vi "Sequence.Compile.vi"(8 "error in (no error)":errorcluster, 11 "State Variables":T1) -> (0 "error out":errorcluster, 2 "output cluster":T3, 3 "State Variables out":T1)   [LabVIEW 2013, in "Simple Sequence Editor.lvlib"]
uses:
  Simple Sequence Editor.lvlib
  Types/StateVariables.ctl
  Types/ChannelProperties.ctl
  Types/Compiled.RTSequenceProperties.ctl
  Types/Compiled.StepProperties.ctl
  Types/Compiled.IOStateProperties.ctl
  Types/Compiled.StepElementProperties.ctl
  Types/StepTypes.ctl
  Types/Compiled.StepCondition.ctl
  Types/OperationTypes.ctl
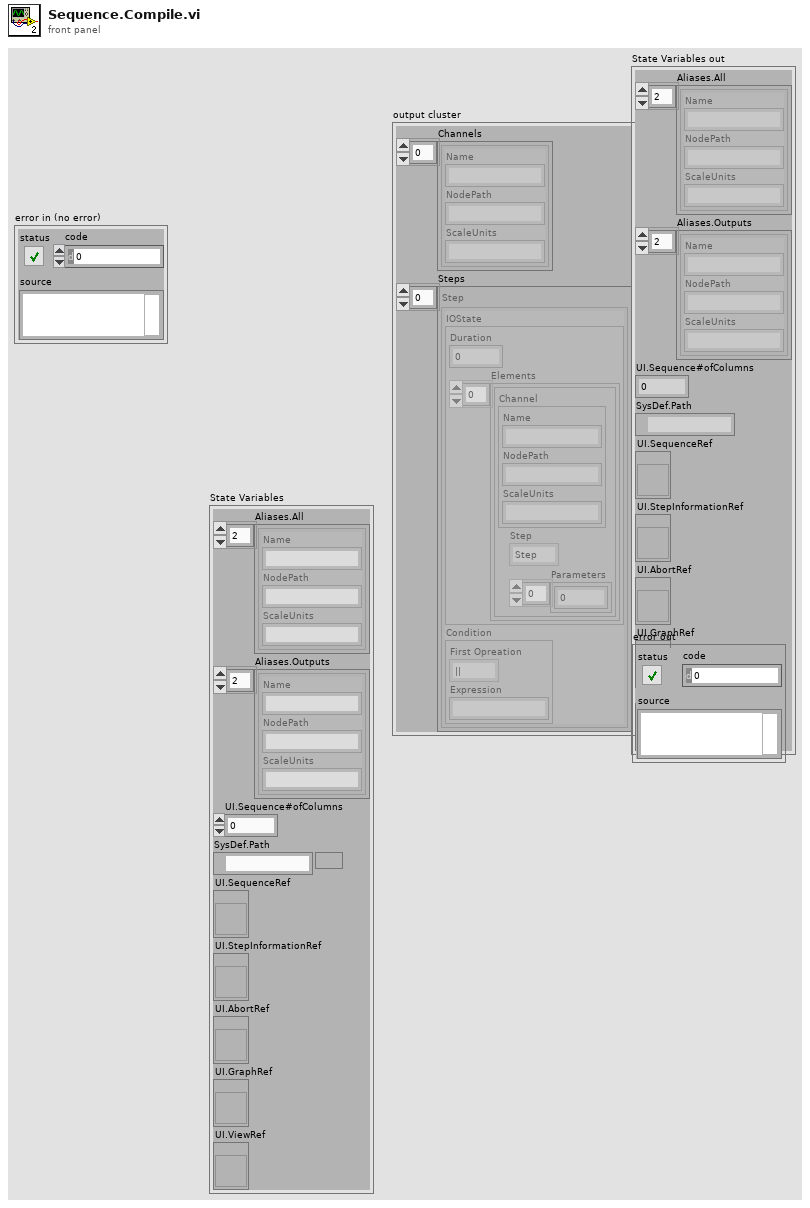
[diagram p1: front panel]
types:
  T1 = typedef "Simple Sequence Editor.lvlib/StateVariables.ctl" = cluster{"Aliases.All":T2[], "Aliases.Outputs":T2[], "UI.Sequence#ofColumns":i32, "SysDef.Path":path, "UI.SequenceRef":refnum<vi>, "UI.StepInformationRef":refnum<vi>, "UI.AbortRef":refnum<vi>, "UI.GraphRef":refnum<vi>, "UI.ViewRef":refnum<vi>}
  T2 = typedef "Simple Sequence Editor.lvlib/ChannelProperties.ctl" = cluster{"Name":string, "NodePath":string, "ScaleUnits":string}
  T3 = typedef "Simple Sequence Editor.lvlib/Compiled.RTSequenceProperties.ctl" = cluster{"Channels":T2[], "Steps":T4[]}
  T4 = typedef "Simple Sequence Editor.lvlib/Compiled.StepProperties.ctl" = cluster{"IOState":T5, "Condition":T8}
  T5 = typedef "Simple Sequence Editor.lvlib/Compiled.IOStateProperties.ctl" = cluster{"Duration":dbl, "Elements":T6[]}
  T6 = typedef "Simple Sequence Editor.lvlib/Compiled.StepElementProperties.ctl" = cluster{"Channel":T2, "Step":T7, "Parameters":dbl[]}
  T7 = typedef "Simple Sequence Editor.lvlib/StepTypes.ctl" = enum8{"Step", "iStep", "Ramp", "Unchanged", "Unknown"}
  T8 = typedef "Simple Sequence Editor.lvlib/Compiled.StepCondition.ctl" = cluster{"First Opreation":T9, "Expression":string}
  T9 = typedef "Simple Sequence Editor.lvlib/OperationTypes.ctl" = enum8{"None", "&&", "||"}
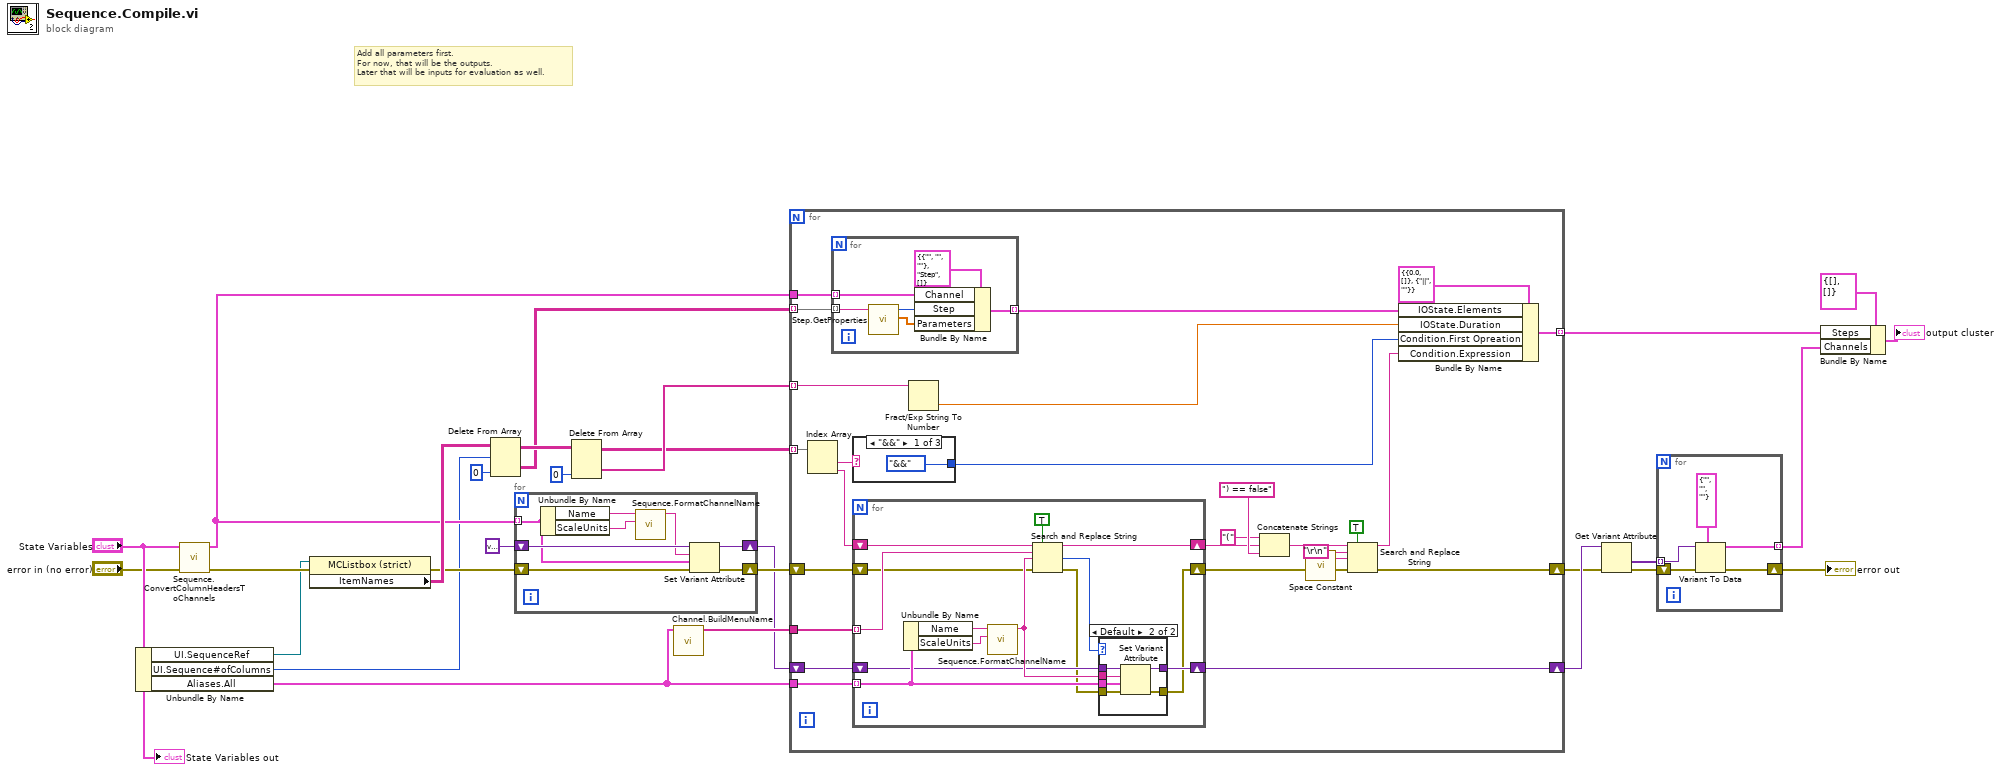
[diagram p0: block diagram]
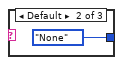
[diagram p3: hidden frame]
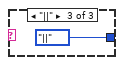
[diagram p4: hidden frame]
diagram:
  # "Add all parameters first.\nFor now, that will be the outputs.\nLater that will be inputs for evaluation as well."
  n1 = Unbundle By Name("State Variables") -> ("UI.SequenceRef"=w2:refnum<vi>, "UI.Sequence#ofColumns"=w1:i32, "Aliases.All"=w17:T2[])
  n2 = call "Sequence.ConvertColumnHeadersToChannels.vi"("error in (no error)"="error in (no error)", "State Variables"="State Variables") -> ("error out"=w3:errorcluster, "Output Channels"=w14:T2[])  [unwired: 8 in]
  n3 = property class="MCListbox (strict)"(reference=w2, error in=w3) -> (error out=w13:errorcluster, "ItemNames"=w25:string[][])  [unwired: 1 out]
  n4 = Delete From Array(array=w25, length=w1, index (col)=0 ("disabled index (col)")) -> (deleted portion=w23:string[][], array with subset deleted=w28:string[][])  [unwired: 1 in]
  n5 = for {
    shift-right: [w35] -> w11
    shift-left: variant ("variant") -> [w36]
    shift-right: [w34] -> w12
    shift-left: w13 -> [w33]
    tunnel: w14 -> [w32] mode=indexing
    n6 = Unbundle By Name(w32) -> ("Name"=w31:string, "ScaleUnits"=w30:string)
    n7 = call "Sequence.FormatChannelName.vi"("ScaleUnits"=w30, "Name"=w31) -> ("String"=w29:string)  [unwired: 9 in]
    n8 = Set Variant Attribute(Variant=w36, name=w29, value=w32, error in=w33) -> (Variant out=w35:variant, error out=w34:errorcluster)  [unwired: 1 out]
  }
  n9 = Delete From Array(array=w28, index (col)=0 ("disabled index (col)")) -> (deleted portion=w24:string[], array with subset deleted=w19:string[][])  [unwired: 2 in]
  n10 = call "Channel.BuildMenuName.vi"("Aliases"=w17) -> ("Aliases Array"=w18:string[])  [unwired: 10 in]
  n11 = for {
    tunnel: w24 -> [w62] mode=indexing
    tunnel: w23 -> [w61] mode=indexing
    tunnel: w14 -> [w60]
    tunnel: [w50] -> w21 mode=indexing
    tunnel: w19 -> [w55] mode=indexing
    tunnel: w18 -> [w54]
    tunnel: w17 -> [w53]
    shift-right: [w44] -> w8
    shift-left: w12 -> [w52]
    shift-right: [w39] -> w10
    shift-left: w11 -> [w40]
    n12 = Index Array(array=w55) -> (element #1=w56:string, element #2=w57:string)  [unwired: 2 in]
    n13 = for {
      tunnel: w61 -> [w93] mode=indexing
      tunnel: w60 -> [w91] mode=indexing
      tunnel: [w88] -> w38 mode=indexing
      n14 = call "Step.GetProperties.vi"("String in"=w93) -> ("Parameters"=w89:dbl[], "Step"=w90:T7)  [unwired: 9 in]
      n15 = Bundle By Name(cluster=T6 {"Channel"={"Name"="", "NodePath"="", "ScaleUnits"=""}, "Step"=enum."Step", "Parameters"=[]}, "Channel"=w91, "Step"=w90, "Parameters"=w89) -> (w88:T6)
    }
    n16 = case shown="\"&&\"" w56 {
      tunnel: [OperationTypes."&&" OperationTypes."None" OperationTypes."||"] -> w41
      frame "&&" {
      }
      frame Default {
      }
      frame "||" {
      }
    }
    n17 = for {
      tunnel: w54 -> [w76] mode=indexing
      tunnel: w53 -> [w70] mode=indexing
      shift-right: [w63] -> w45
      shift-left: w52 -> [w67]
      shift-right: [w71] -> w58
      shift-left: w57 -> [w75]
      shift-right: [w68] -> w39
      shift-left: w40 -> [w65]
      n18 = Unbundle By Name(w70) -> ("Name"=w73:string, "ScaleUnits"=w74:string)
      n19 = call "Sequence.FormatChannelName.vi"("ScaleUnits"=w74, "Name"=w73) -> ("String"=w69:string)  [unwired: 9 in]
      n20 = Search and Replace String(replace all?=TRUE ("replace all? (F)"), input string=w75, search string=w76, replace string=w69, error in=w67) -> (result string=w71:string, number of replacements=w66:i32, error out=w64:errorcluster)  [unwired: 3 in, 1 out]
      n21 = case shown="Default" w66 {
        tunnel: w70 -> [_ w84]
        tunnel: w69 -> [_ w83]
        tunnel: [w78 w82] -> w68
        tunnel: w65 -> [w78 w81]
        tunnel: w64 -> [w77 w80]
        tunnel: [w77 w79] -> w63
        frame -1, 0 {
        }
        frame Default {
          n22 = Set Variant Attribute(Variant=w81, name=w83, value=w84, error in=w80) -> (Variant out=w82:variant, error out=w79:errorcluster)  [unwired: 1 out]
        }
      }
    }
    n23 = Fract/Exp String To Number(string=w62) -> (number=w37:dbl)  [unwired: 3 in, 1 out]
    n24 = Concatenate Strings("(" ("string"), w58, ") == false" ("string")) -> (w48:string)
    n25 = call <vilib>:"Space Constant.vi"() -> ("String"=w46:string)
    n26 = Search and Replace String(replace all?=TRUE ("replace all? (F)"), input string=w48, search string="\r\n", replace string=w46, error in=w45) -> (result string=w42:string, error out=w44:errorcluster)  [unwired: 3 in, 2 out]
    n27 = Bundle By Name(cluster=T4 {"IOState"={"Duration"=0.0, "Elements"=[]}, "Condition"={"First Opreation"=enum."||", "Expression"=""}} ("Step"), "IOState.Elements"=w38, "IOState.Duration"=w37, "Condition.First Opreation"=w41, "Condition.Expression"=w42) -> (w50:T4)
  }
  n28 = Get Variant Attribute(Variant=w10, error in=w8) -> (values=w9:variant[], error out=w7:errorcluster)  [unwired: 2 in, 2 out]
  n29 = for {
    tunnel: w9 -> [w98] mode=indexing
    shift-right: [w96] -> w5
    shift-left: w7 -> [w97]
    tunnel: [w94] -> w6 mode=indexing
    n30 = Variant To Data(error in=w97, type=T2 {"Name"="", "NodePath"="", "ScaleUnits"=""} ("cluster"), Variant=w98) -> (data=w94:T2, error out=w96:errorcluster)
  }
  "error out" <- w5
  n31 = Bundle By Name(cluster=T3 {"Channels"=[], "Steps"=[]}, "Steps"=w21, "Channels"=w6) -> (→"output cluster":T3)
  "State Variables out" <- "State Variables"
